vi "测试状态判断.vi"(11 "TimingControl 输入":refnum<class "TimingControl.lvclass">) -> (2 "数据":cluster{"启动":bool, "控制命令":T1, "测量参数":T2}, 3 "TimingControl 输出":refnum<class "TimingControl.lvclass">)   [LabVIEW 2016, in "TimingControl.lvlib" / "TimingControl.lvclass"]
uses:
  TimingControl.lvclass
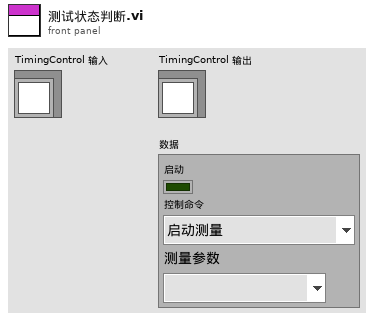
[diagram p1: front panel]
types:
  T1 = typedef "TimingControl.lvlib/TimingControl.lvclass/国标控制命令.ctl" = enum16{"启动测量", "标样核查", "零点核查", "跨度核查", "空白测试", "平行样测试", "加标回收", "空白校准", "标样校准", "初始化（清洗）", "停止测试", "仪器重启", "校时", "模式设置", "测量间隔设置"}
  T2 = typedef "TimingControl.lvlib/TimingControl.lvclass/测量参数.ctl" = u16
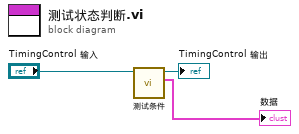
[diagram p0: block diagram]
diagram:
  n1 = call "测试条件.vi"("TimingControl 输入"="TimingControl 输入") -> ("簇"=→"数据":cluster{bool, "控制命令":T1, "测量参数":T2}, "TimingControl 输出"=→"TimingControl 输出":refnum<class "TimingControl.lvclass">)  [unwired: 9 in]
